vi "SysDef.Search.Name.vi"(8 "error in (no error)":errorcluster, 10 "Name":string, 11 "nodeID":u64) -> (0 "error out":errorcluster, 1 "Value out":u64, 3 "nodeID out":u64, 4 "Found?":bool)   [LabVIEW 2027, in "Advanced System Definition.lvlib"]
uses:
  SysDef API/Advanced System Definition.lvlib
  <vilib>/NI VeriStand/Custom Device Tools/Custom Device Utility Library/NI VeriStand - Search for Item by Name.vi
  C:/NetCore/niveristand-custom-device-development-tools/advanced-sysdef-api/Source/_SubVIs/SysDef.Search.Name.vi/NationalInstruments.VeriStand.SystemDefinitionAPI
  NationalInstruments.VeriStand.SystemDefinitionAPI
  C:/NetCore/niveristand-custom-device-development-tools/advanced-sysdef-api/Source/_SubVIs/SysDef.Search.Name.vi/NationalInstruments.VeriStand.SystemStorage
  NationalInstruments.VeriStand.SystemStorage
  <vilib>/NI VeriStand/Custom Device Tools/Custom Device Utility Library/Custom Device Utility Library.lvlib
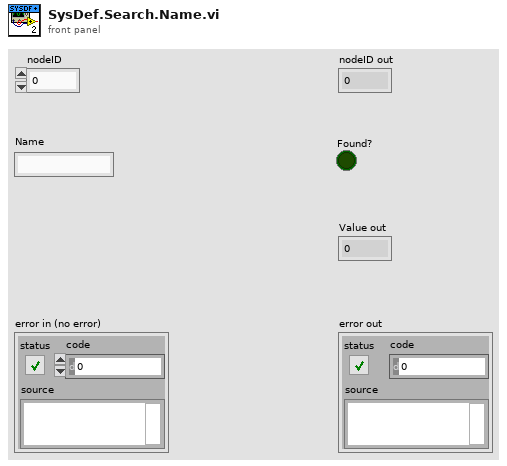
[diagram p1: front panel]
types:
  T1 = typedef "Custom Device API.lvlib/Custom Device Item Ref.ctl" = u64
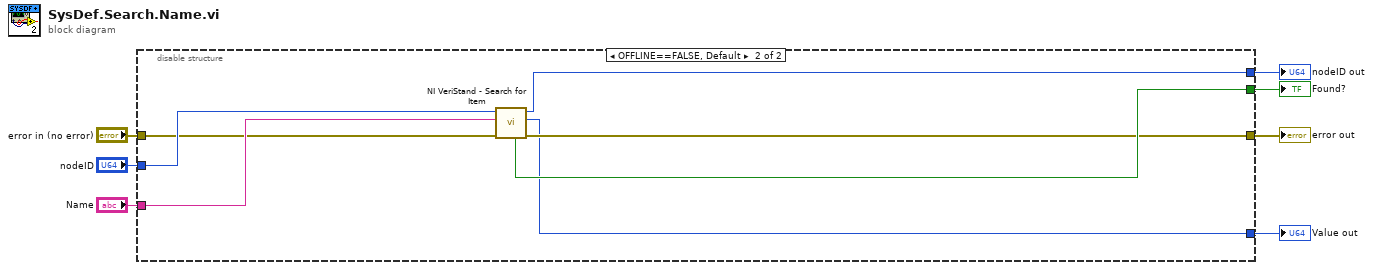
[diagram p0: block diagram]
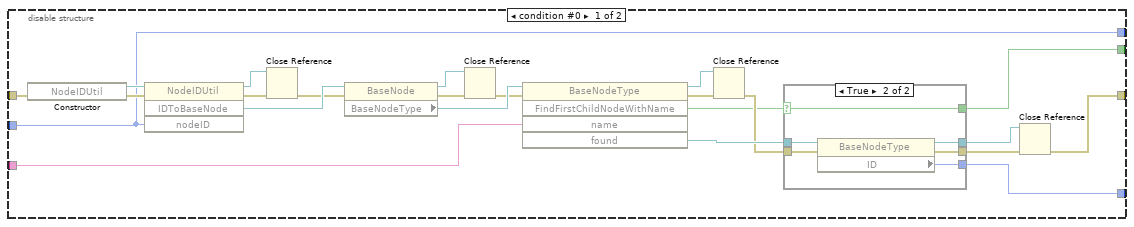
[diagram p2: hidden frame]
diagram:
  n1 = disable-structure shown="OFFLINE==FALSE, Default" {
    disable-tunnel: "error in (no error)" -> [w24 w44]
    disable-tunnel: "nodeID" -> [w21 w45]
    disable-tunnel: [w10 w42] -> w5
    disable-tunnel: "Name" -> [w17 w46]
    disable-tunnel: [w8 w43] -> w3
    disable-tunnel: [w14 w40] -> w2
    disable-tunnel: [w21 w41] -> w1
    frame condition #0 {
      n2 = constructor class="NodeIDUtil"(error in=w24) -> (reference out=w30:refnum<k24>, error out=w29:errorcluster)  [unwired: 2 in, 1 out]
      n3 = invoke class="NodeIDUtil" method="IDToBaseNode"(reference=w30, error in=w29, "nodeID"=w21) -> (reference out=w25:refnum<k24>, error out=w27:errorcluster, "IDToBaseNode"=w28:refnum<k24>)  [unwired: 1 in, 1 out]
      n4 = Close Reference(reference=w25, error in (no error)=w27) -> (error out=w26:errorcluster)
      n5 = property class="BaseNode"(reference=w28, error in=w26) -> (reference out=w23:refnum<k24>, error out=w22:errorcluster, "BaseNodeType"=w20:refnum<k24>)
      n6 = Close Reference(reference=w23, error in (no error)=w22) -> (error out=w19:errorcluster)
      n7 = invoke class="BaseNodeType" method="FindFirstChildNodeWithName"(reference=w20, error in=w19, "name"=w17) -> (reference out=w16:refnum<k24>, error out=w18:errorcluster, "FindFirstChildNodeWithName"=w9:bool, "found"=w15:refnum<k24>)  [unwired: 2 in, 1 out]
      n8 = Close Reference(reference=w16, error in (no error)=w18) -> (error out=w13:errorcluster)
      n9 = case shown="True" w9 {
        selector: w9 -> [w33 w34]
        tunnel: w15 -> [w32 w39]
        tunnel: [_ w38] -> w14
        tunnel: w13 -> [w31 w37]
        tunnel: [w32 w36] -> w12
        tunnel: [w31 w35] -> w11
        tunnel: [w33 w34] -> w8
        frame False {
        }
        frame True {
          n10 = property class="BaseNodeType"(reference=w39, error in=w37) -> (reference out=w36:refnum<k24>, error out=w35:errorcluster, "ID"=w38:u64)
        }
      }
      n11 = Close Reference(reference=w12, error in (no error)=w11) -> (error out=w10:errorcluster)
    }
    frame condition #1 (active) {
      n12 = call-poly <vilib>:"NI VeriStand - Search for Item.vi"("error in"=w44, "Item Name"=w46, "Section Ref in"=w45) -> ("error out"=w42:errorcluster, "Item Ref"=w40:T1, "Section Ref out"=w41:T1, "Found"=w43:bool)  [unwired: 5 in]
    }
  }
  "nodeID out" <- w1
  "error out" <- w5
  "Value out" <- w2
  "Found?" <- w3
